vi "Set Timeout.vi"(8 "error in (no error)":errorcluster, 10 "Milliseconds To Wait (-1, forever)":i32=-1, 11 "State Actor in":refnum<class "State Actor.lvclass">) -> (0 "error out":errorcluster, 3 "State Actor out":refnum<class "State Actor.lvclass">)   [LabVIEW 2024, in "State Actor.lvlib" / "State Actor.lvclass"]
uses:
  State Actor.lvclass
  C:/Program Files (x86)/National Instruments/LabVIEW 2024/vi.lib/ActorFramework/Actor/Actor.lvclass
  State Actor Messages/Timeout Msg/Timeout Msg.lvclass
  C:/Program Files (x86)/National Instruments/LabVIEW 2024/vi.lib/ActorFramework/Message/Message.lvclass
  <vilib>/ActorFramework/Message Enqueuer/Message Priority.ctl
  <vilib>/ActorFramework/Actor/Actor.lvclass/Actor.ctl
  <vilib>/ActorFramework/Message Enqueuer/Message Enqueuer.lvclass/Message Enqueuer.ctl
  State Actor.lvclass/State Actor.ctl
  <vilib>/ActorFramework/Message Enqueuer/Init from Existing Queue.vi
  <vilib>/ActorFramework/Message Enqueuer/Message Enqueuer.lvclass
  <vilib>/ActorFramework/Actor/Actor.lvclass
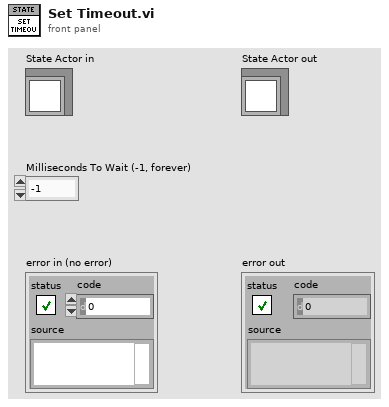
[diagram p1: front panel]
types:
  T1 = typedef "Actor Framework.lvlib/Message Enqueuer.lvclass/Message Priority.ctl" = enum16{"Low", "Normal", "High"}
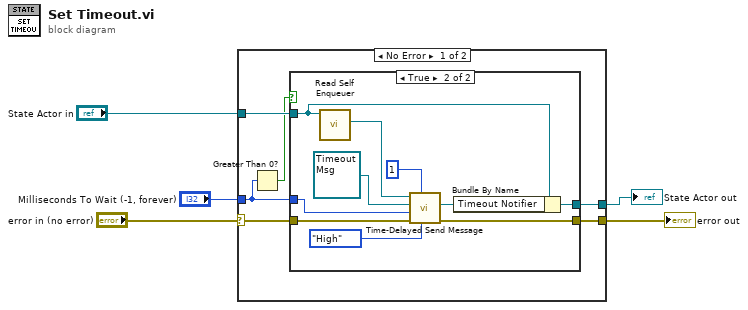
[diagram p0: block diagram]
diagram:
  n1 = case shown="No Error" "error in (no error)" {
    selector: "error in (no error)" -> [w10 w25]
    tunnel: [w9 w25] -> w4
    tunnel: [w6 w24] -> w2
    tunnel: "State Actor in" -> [w11 w24]
    tunnel: "Milliseconds To Wait (-1, forever)" -> [w7 _]
    frame No Error {
      n2 = Greater Than 0?(x=w7) -> (x > 0?=w8:bool)
      n3 = case shown="True" w8 {
        tunnel: w11 -> [w12 w16]
        tunnel: w10 -> [w13 w21]
        tunnel: [w13 w20] -> w9
        tunnel: w7 -> [_ w17]
        tunnel: [w12 w14] -> w6
        frame False {
        }
        frame True {
          n4 = call <vilib>:"Read Self Enqueuer.vi"("Actor"=w16) -> ("Self Enqueuer"=w23:refnum<class "Message Enqueuer.lvclass">)  [unwired: 10 in]
          n5 = call <vilib>:"Time-Delayed Send Message.vi"("Message Priority (Normal)"=Message_Priority."High", "# Copies (0 = infinite repeat)"=u32 1, "error in (no error)"=w21, "Milliseconds To Wait"=w17, "Message"=refnum<class "Timeout Msg.lvclass"> refnum ("State Actor.lvlib:Timeout Msg.lvclass"), "Message Enqueuer"=w23) -> ("error out"=w20:errorcluster, "Delivery Notifier"=w15:refnum<notifier>)  [unwired: 4 in]
          n6 = Bundle By Name(cluster=w16, "Timeout Notifier"=w15) -> (w14:refnum<class "State Actor.lvclass">)
        }
      }
    }
    frame Error {
    }
  }
  "error out" <- w4
  "State Actor out" <- w2
